vi "main.vi"() -> ()   [LabVIEW 2017]
panel:
  out "Result String":string
  out "Numeric":i32
  out "elapsed time":dbl
  in  "?":bool
  in  "?":bool
  in  "?":bool
  out "Message":string
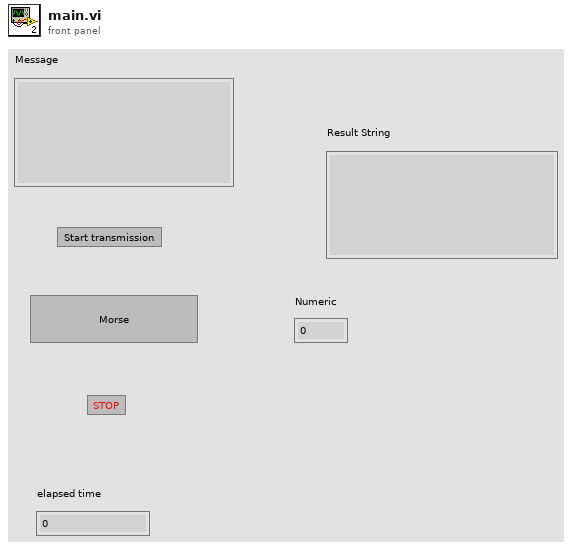
[diagram p1: front panel]
types:
  T1 = enum16{"StartScreen", "StartTick", "StopTick", "EvaluateSign"}
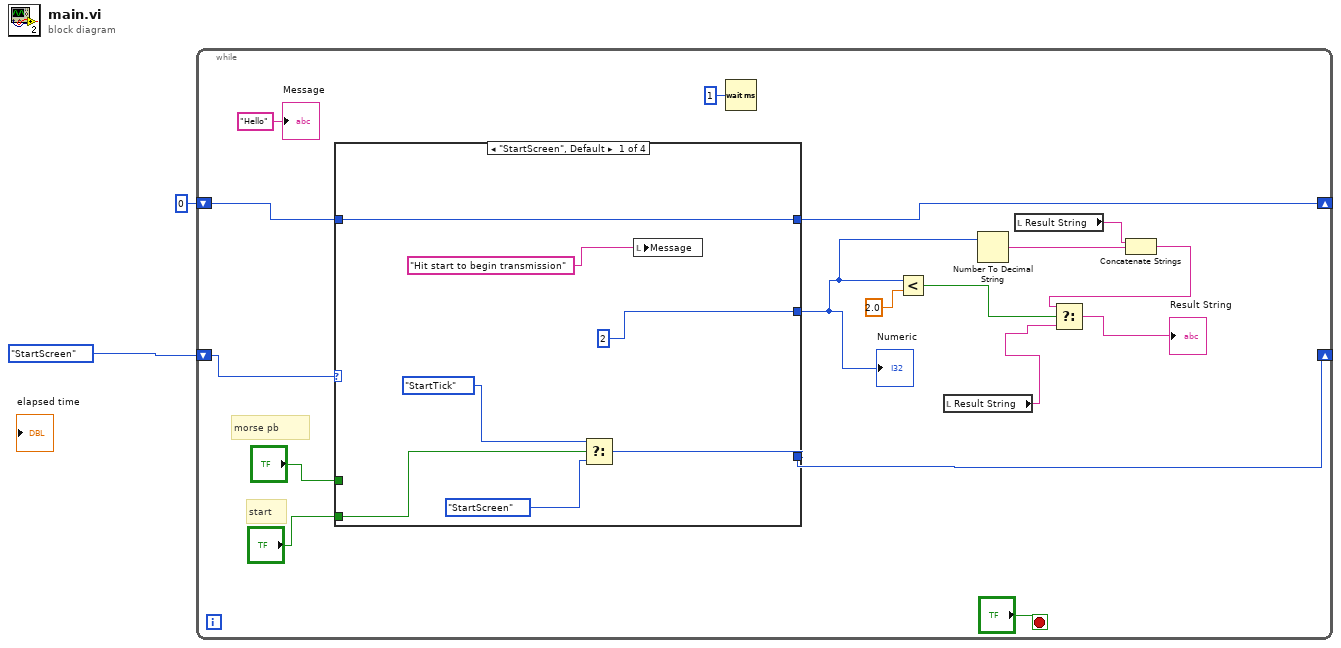
[diagram p0: block diagram]
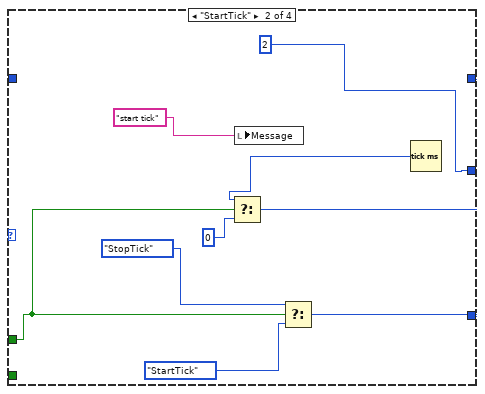
[diagram p2: hidden frame]
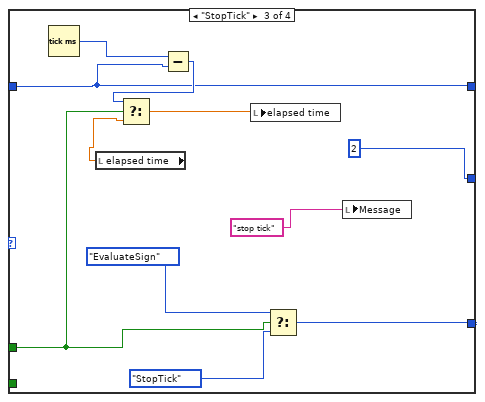
[diagram p3: hidden frame]
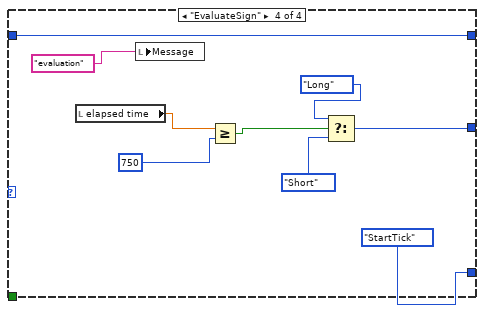
[diagram p4: hidden frame]
diagram:
  n1 = while {
    shift-right: [w15] -> _
    shift-left: T1."StartScreen" -> [w16]
    shift-right: [w12] -> _
    shift-left: u32 0 ("millisecond timer value") -> [w11]
    stop <- "?" stop-if-true
    # "start"
    # "morse pb"
    n2 = case shown="\"StartScreen\", Default" w16 {
      tunnel: [w23 w32 w45 T1."StartTick"] -> w15
      tunnel: "?" -> [_ w31 w42 _]
      tunnel: "?" -> [w22 _ _ _]
      tunnel: [w21 w28 w37 w54] -> w12
      tunnel: w11 -> [w21 _ w37 w54]
      tunnel: [2 2 2 w47] -> w6
      frame "StartScreen", Default {
        n3 = Select(t=T1."StartTick", s=w22, f=T1."StartScreen") -> (s? t:f=w23:T1)
        n4 = local write "Message"("Hit start to begin transmission" ("Message")) -> ()
      }
      frame "StartTick" {
        n5 = local write "Message"("start tick" ("Message")) -> ()
        n6 = Select(t=T1."StopTick", s=w31, f=T1."StartTick") -> (s? t:f=w32:T1)
        n7 = Tick Count (ms)() -> (millisecond timer value=w29:u32)
        n8 = Select(t=w29, s=w31, f=u32 0) -> (s? t:f=w28:u32)
      }
      frame "StopTick" {
        n9 = Tick Count (ms)() -> (millisecond timer value=w40:u32)
        n10 = local read "elapsed time"() -> (w38:dbl)
        n11 = Subtract(x=w40, y=w37) -> (x-y=w39:u32)
        n12 = Select(t=w39, s=w42, f=w38) -> (s? t:f=w41:dbl)
        n13 = local write "elapsed time"(w41) -> ()
        n14 = Select(t=T1."EvaluateSign", s=w42, f=T1."StopTick") -> (s? t:f=w45:T1)
        n15 = local write "Message"("stop tick" ("Message")) -> ()
      }
      frame "EvaluateSign" {
        n16 = local read "elapsed time"() -> (w53:dbl)
        n17 = local write "Message"("evaluation" ("Message")) -> ()
        n18 = Greater Or Equal?(x=w53, y=750) -> (x >= y?=w50:bool)
        n19 = Select(t=enum16{"Short", "Long", "No update"}."Long", s=w50, f=enum16{"Short", "Long", "No update"}."Short") -> (s? t:f=w47:enum16{"Short", "Long", "No update"})
      }
    }
    "Numeric" <- w6
    n20 = Wait (ms)(milliseconds to wait=u32 1) -> ()  [unwired: 1 out]
    n21 = Less?(x=w6, y=2.0) -> (x < y?=w10:bool)
    n22 = local read "Result String"() -> (w7:string)
    n23 = Number To Decimal String(number=w6) -> (decimal integer string=w3:string)  [unwired: 1 in]
    n24 = local read "Result String"() -> (w4:string)
    n25 = Concatenate Strings(w4, w3) -> (w5:string)
    n26 = Select(t=w5, s=w10, f=w7) -> (s? t:f=→"Result String":string)
    "Message" <- "Hello" ("Message")
  }
